vi "Source_Combo box controls ini setup.vi"() -> (0 "error out":errorcluster, 2 "Keys setup":T1, 5 "Section name":string)   [LabVIEW 2017]
uses:
  Configuration code/Typedefs/Ini file interface (String).ctl
  Global Variables/gl_UI Ctrl Refs.vi
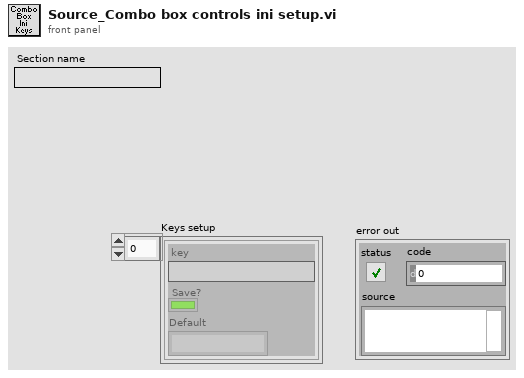
[diagram p1: front panel]
types:
  T1 = typedef "Ini file interface (String).ctl" = cluster{"key":string, "Save?":bool, "Default":string}[]
  T2 = cluster{"key":string, "Save?":bool, "Default":string}
  T3 = typedef "UI ctrl refs cluster.ctl" = cluster{"Top level VI path":path, "Top level VI ref":refnum<vi>, "User menu ref":refnum<k9>, "Sub Panel control":refnum<vi>, "Imaging Param Tab":refnum<vi>, "Occurrence-Start drivers":refnum<k4>, "Occurrence-Speed logging initialised":refnum<k4>, "Occurrence-XYZ stage initialised":refnum<k4>, "Exit button":refnum<vi>, "Status ind":refnum<vi>, "Set as origin":refnum<vi>, "Speed Logging":refnum<vi>, "Time Lapse":refnum<vi>, "Live Imaging":refnum<vi>, "AOL Z Stack":refnum<vi>, "Motor Z Stack":refnum<vi>, "Funct Acq button":refnum<vi>, "Hard Shutter":refnum<vi>, "Virtual Shutter":refnum<vi>, "Laser Power":refnum<vi>, "AOL Mode":refnum<vi>, "Frame Size":refnum<vi>, "Field of View":refnum<vi>, "Dwell Time":refnum<vi>, "Zoom":refnum<vi>, "AOL Z":refnum<vi>, "Objective":refnum<vi>, "Axis":refnum<vi>, "Paths & Names":refnum<vi>, "Experiment folder path (ind.)":refnum<vi>, "Last State (Ind.)":refnum<vi>, "Laser wavelength ind (nm)":refnum<vi>, "Averages":refnum<vi>, "Angle (degrees)":refnum<vi>, "X centre":refnum<vi>, "Y centre":refnum<vi>, "Plane Mode":refnum<vi>, "# Planes":refnum<vi>, "Z Start":refnum<vi>, "Z Stop":refnum<vi>, "Z Step":refnum<vi>, "PMT 1":refnum<vi>, "PMT 2":refnum<vi>, "Stage XYZ Position":refnum<vi>, "Pockels@Z Start":refnum<vi>, "Pockels@Z Stop":refnum<vi>, "Obtain Z Start":refnum<vi>, "Obtain Z Stop":refnum<vi>, "Live stim.trig.period":refnum<vi>, "Live stim.trig.enable":refnum<vi>, "Movement Correction":refnum<vi>, "Load Reference Image":refnum<vi>, "XY Stage Move":refnum<vi>, "MovCor Cluster":refnum<vi>, "RefDAQParam":refnum<vi>, "Funct. Acq. Pockels Modulation":refnum<vi>, "Background MovCor":refnum<vi>, "Ref Laser Power":refnum<vi>, "Enable Video Recording":refnum<vi>, "Video Record-Live Imaging":refnum<vi>, "Video Record-Funct acq":refnum<vi>, "Reference Source":refnum<vi>, "AOL Z-stack Chirps Ready (ind)":refnum<vi>, "Target time between mov.cor. ref triggers (ms)":refnum<vi>, "Funct. Acq. Ref frame save":refnum<vi>, "Tracking button":refnum<vi>, "Show ref plots window":refnum<vi>, "Center freq ind (nm)":refnum<vi>, "Pickup mode (ind)":refnum<vi>, "Logging queue (ind)":refnum<vi>, "Back aperture power (ind.)":refnum<vi>, "Power after objective (ind.)":refnum<vi>, "Switch user":refnum<vi>}
  T4 = cluster{"key":string, "Save?":bool, "Default":string}[]
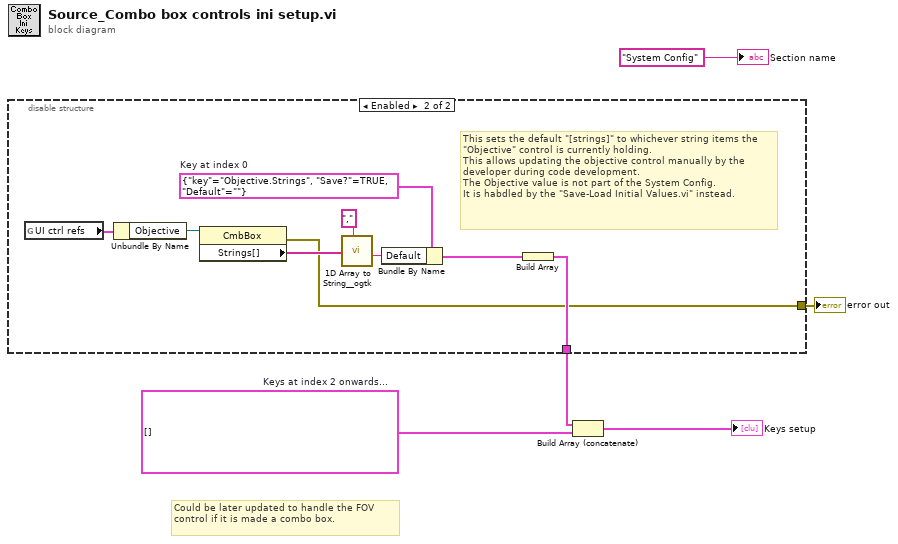
[diagram p0: block diagram]
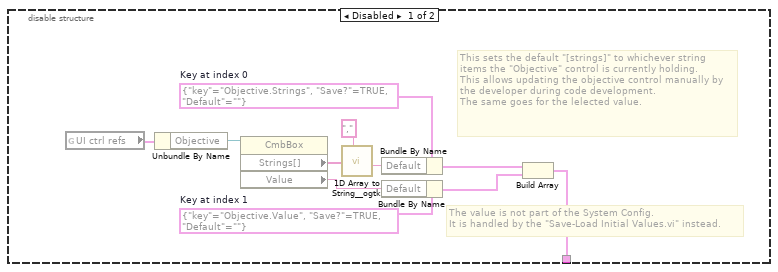
[diagram p2: hidden frame]
diagram:
  w4 = T1 []  # Keys at index 2 onwards...
  # "Could be later updated to handle the FOV control if it is made a combo box."
  n1 = disable-structure shown="Enabled" {
    disable-tunnel: [w9 w18] -> w2
    disable-tunnel: [_ w17] -> w1
    frame Disabled {
      w7 = T2 {"key"="Objective.Value", "Save?"=TRUE, "Default"=""}  # Key at index 1
      w12 = T2 {"key"="Objective.Strings", "Save?"=TRUE, "Default"=""}  # Key at index 0
      # "The value is not part of the System Config.\nIt is handled by the \"Save-Load Initial Values.vi\" instead."
      # "This sets the default \"[strings]\" to whichever string items the \"Objective\" control is currently holding.\nThis allows updating the objective control manually by the developer during code development.\nThe same goes for the lelected value."
      n2 = global read "gl_UI Ctrl Refs.vi" "UI ctrl refs"() -> (w16:T3)
      n3 = Unbundle By Name(w16) -> ("Objective"=w13:refnum<vi>)
      n4 = property class="CmbBox"(reference=w13) -> ("Strings[]"=w14:string[], "Value"=w8:string)  [unwired: 1 in, 2 out]
      n5 = call <userlib>:"1D Array to String__ogtk.vi"("delimiter (Tab)"=",", "Array of Strings"=w14) -> ("delimited string"=w11:string)  [unwired: 9 in]
      n6 = Bundle By Name(cluster=w12, "Default"=w11) -> (w10:T2)
      n7 = Bundle By Name(cluster=w7, "Default"=w8) -> (w6:T2)
      n8 = Build Array(w10, w6) -> (w9:T4)
    }
    frame Enabled {
      w21 = T2 {"key"="Objective.Strings", "Save?"=TRUE, "Default"=""}  # Key at index 0
      # "This sets the default \"[strings]\" to whichever string items the \"Objective\" control is currently holding.\nThis allows updating the objective control manually by the developer during code development.\nThe Objective value is not part of the System Config.\nIt is habdled by the \"Save-Load Initial Values.vi\" instead."
      n9 = global read "gl_UI Ctrl Refs.vi" "UI ctrl refs"() -> (w25:T3)
      n10 = Unbundle By Name(w25) -> ("Objective"=w22:refnum<vi>)
      n11 = property class="CmbBox"(reference=w22) -> (error out=w17:errorcluster, "Strings[]"=w23:string[])  [unwired: 1 in, 1 out]
      n12 = call <userlib>:"1D Array to String__ogtk.vi"("delimiter (Tab)"=",", "Array of Strings"=w23) -> ("delimited string"=w20:string)  [unwired: 9 in]
      n13 = Bundle By Name(cluster=w21, "Default"=w20) -> (w19:T2)
      n14 = Build Array(w19) -> (w18:T4)
    }
  }
  "error out" <- w1
  n15 = Build Array (concatenate)(w2, w4) -> (→"Keys setup":T1)
  "Section name" <- "System Config" ("key")
